vi "Generate Scan.vi"(8 "error in (no error)":errorcluster, 11 "Galvo in":refnum<class "Galvo.lvclass">) -> (0 "error out":errorcluster, 3 "Galvo out":refnum<class "Galvo.lvclass">)   [LabVIEW 2014, in "Galvo.lvclass"]
uses:
  Galvo.lvclass
  Galvo.lvclass/Galvo.ctl
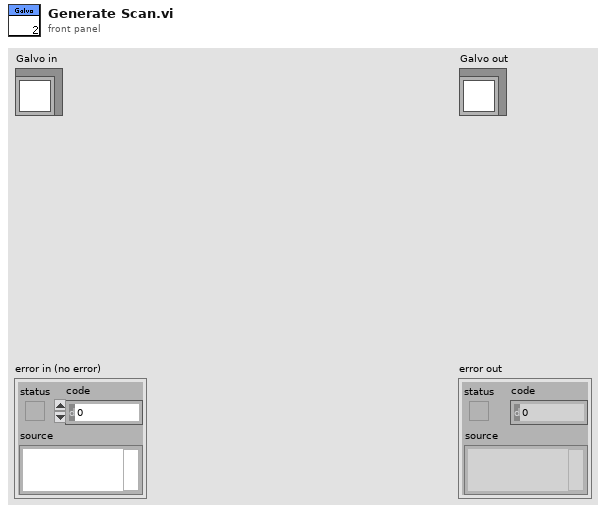
[diagram p1: front panel]
types:
  T1 = typedef "Galvo.lvclass/Scanning Cluster.ctl" = cluster{"Fast Axis Offset":sgl, "Slow Axis Offset":sgl, "Slow Axis Amp":sgl, "Fast Axis Amp":sgl, "Scan Pattern":enum16{"Raster"}}
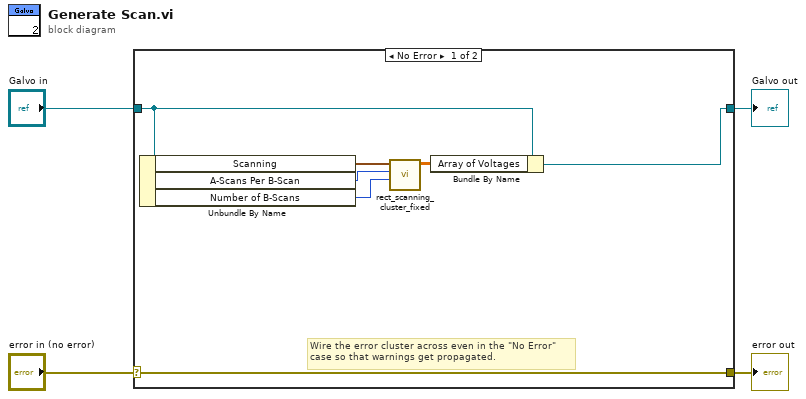
[diagram p0: block diagram]
diagram:
  n1 = case shown="No Error" "error in (no error)" {
    selector: "error in (no error)" -> [w11 w13]
    tunnel: [w11 w13] -> w3
    tunnel: [w7 w12] -> w1
    tunnel: "Galvo in" -> [w8 w12]
    frame No Error {
      # "Wire the error cluster across even in the \"No Error\"\ncase so that warnings get propagated."
      n2 = Unbundle By Name(w8) -> ("Scanning"=w10:T1, "A-Scans Per B-Scan"=w6:u32, "Number of B-Scans"=w5:u32)
      n3 = call "rect_scanning_cluster_fixed.vi"("Slow Axis"=w5, "Fast Axis"=w6, "Scanning"=w10) -> ("Scan Pattern 7"=w9:dbl[][])  [unwired: 8 in]
      n4 = Bundle By Name(cluster=w8, "Array of Voltages"=w9) -> (w7:refnum<class "Galvo.lvclass">)
    }
    frame Error {
    }
  }
  "error out" <- w3
  "Galvo out" <- w1
